vi "Get_Position_Info.vi"(2 "Analysis Info cluster":T1[](array[typedef]) {"Sync Delay Time (s)" format="%.4f"; "Total Meas Time (s)" format="%_5g"; "Sd Error in Variance" format="%_3g"; "Skew_u" format="%_3g"; "% u'/U" format="%_3g"; "Sd Error in Mean" format="%_3g"; "Kurt_u" format="%_3g"; "u^4" format="%_3g"; "u^3" format="%_3g"; "U" format="%_3g"; "u^2" format="%_3g"}, 3 "Setup file string":string) -> (0 "Analysis Info cluster 2":T1[](array[typedef]) {"Sync Delay Time (s)" format="%.4f"; "Total Meas Time (s)" format="%_5g"; "Sd Error in Variance" format="%_3g"; "Skew_u" format="%_3g"; "% u'/U" format="%_3g"; "Sd Error in Mean" format="%_3g"; "Kurt_u" format="%_3g"; "u^4" format="%_3g"; "u^3" format="%_3g"; "U" format="%_3g"; "u^2" format="%_3g"})   [LabVIEW 2021]
uses:
  Controls/Analysis_info_cluster.ctl
  Controls/Inst_type.ctl
  Controls/Instrument_Array.ctl
  Controls/User_Specific_mode.ctl
  Globals/Meas_global.vi
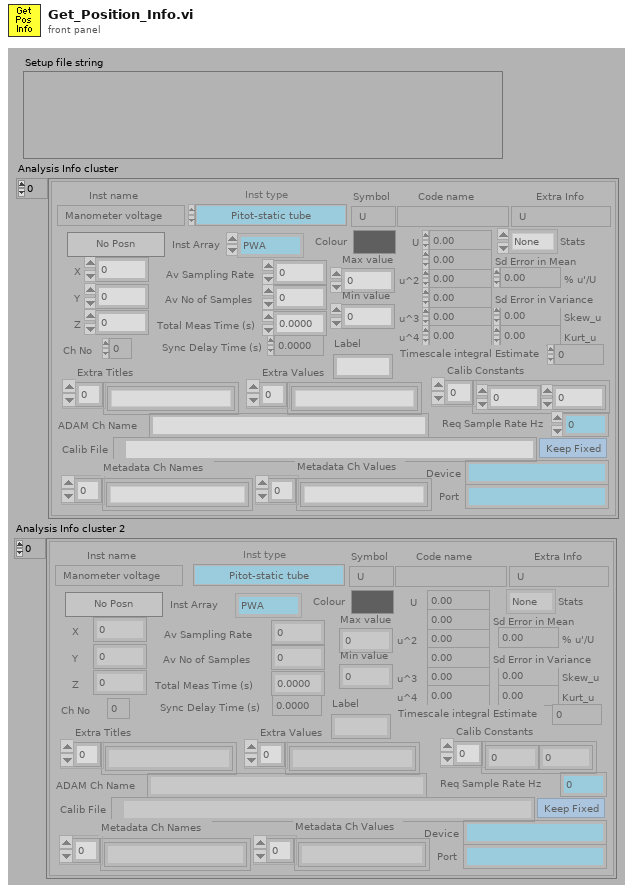
[diagram p1: front panel]
types:
  T1 = typedef "Analysis_info_cluster.ctl" = cluster{"Colour":u32, "Inst type":T2, "Inst name":string, "Symbol":string, "Code name":string, "Extra Info":string, "Inst Array":T3, "Extra Titles":string[], "Extra Values":string[], "U":dbl, "u^2":dbl, "u^3":dbl, "u^4":dbl, "Skew_u":dbl, "Kurt_u":dbl, "Sd Error in Mean":dbl, "% u'/U":dbl, "X":dbl, "Y":dbl, "Z":dbl, "Timescale integral Estimate":dbl, "Sd Error in Variance":dbl, "Calib File":path, "Calib Constants":dbl[], "Output Position":bool, "Stats":enum16{"None", "Basic", "Full"}, "Av Sampling Rate":dbl, "Av No of Samples":dbl, "Total Meas Time (s)":dbl, "ADAM Ch Name":string, "Max value":dbl, "Min value":dbl, "Req Sample Rate Hz":dbl, "Sync Delay Time (s)":dbl, "Ch No":i16, "Device":string, "Use Latest Calib":bool, "Port":string, "Metadata Ch Names":string[], "Metadata Ch Values":string[], "Label":string}
  T2 = typedef "Inst_type.ctl" = enum16{"Raw voltage", "Raw with zero offsetting", "Propeller anemometer", "Pressure Transducer", "Pitot-static tube", "Hot wire", "Cross wire 1", "Cross wire 2", "Generic Linear", "Generic Polynomial", "Generic BackPoly", "Fast FID", "Thermocouple", "Cold wire", "Pulsed Wire", "LDA Vel", "LDA Tran time", "LDA Arr time", "Microphone"}
  T3 = typedef "Instrument_Array.ctl" = enum16{"PWA", "LDA", "Analogue"}
  T4 = typedef "Initial Positions.ctl" = cluster{"Initial XYZ":dbl[], "Traverse Setup":string, "On Axes":string, "Identity String":string}
  T5 = typedef "Post_Process.ctl" = enum16{"Take New Data", "Post Process Raw Data File"}
  T6 = typedef "User_Specific_mode.ctl" = enum16{"Check VI only", "Run VI"}
  T7 = cluster{"Initial XYZ[0]":dbl, "Initial XYZ[1]":dbl, "Initial XYZ[2]":dbl}
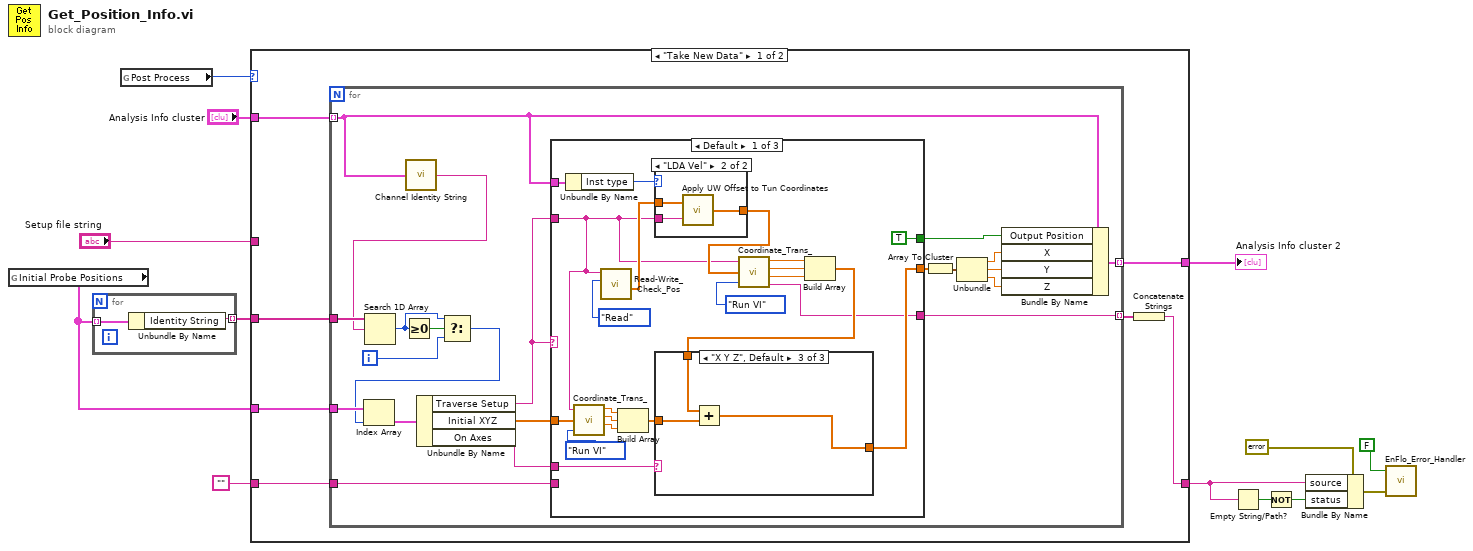
[diagram p0: block diagram]
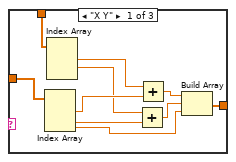
[diagram p3: hidden frame]
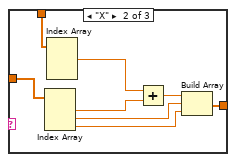
[diagram p4: hidden frame]
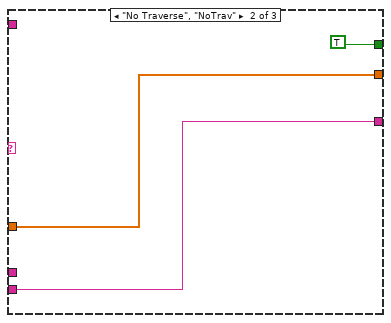
[diagram p5: hidden frame]
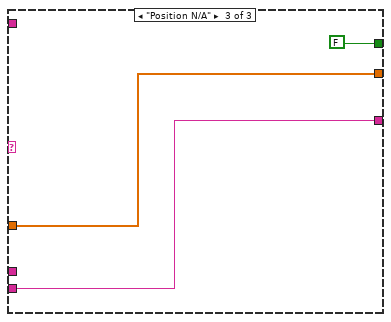
[diagram p6: hidden frame]
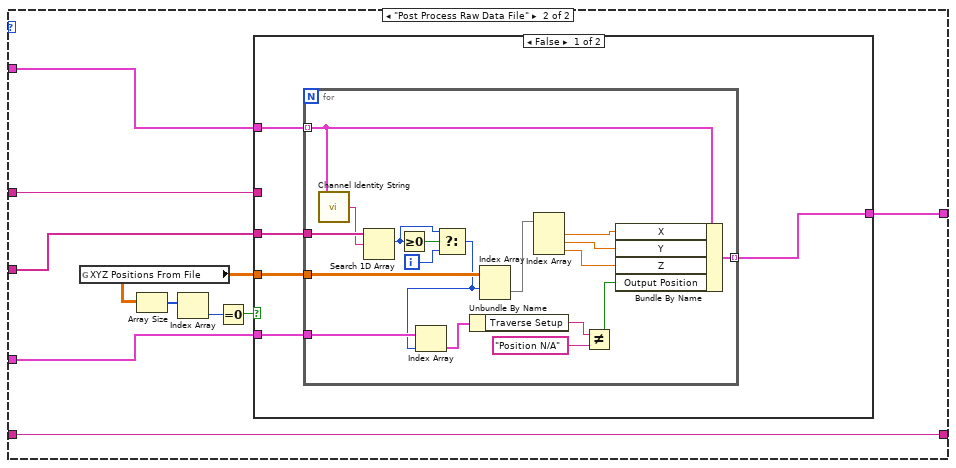
[diagram p7: hidden frame]
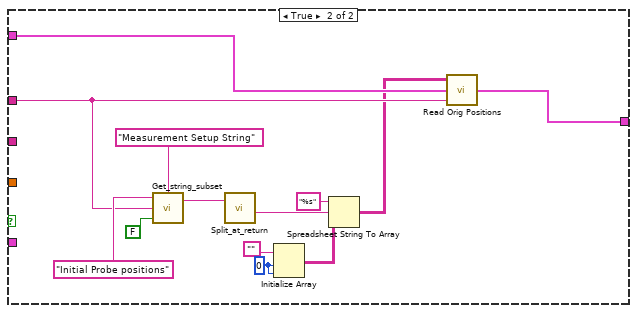
[diagram p8: hidden frame]
diagram:
  n1 = global read "Meas_global.vi" "Initial Probe Positions"() -> (w2:T4[])
  n2 = for {
    tunnel: [w15] -> w1 mode=indexing
    tunnel: w2 -> [w14] mode=indexing
    n3 = Unbundle By Name(w14) -> ("Identity String"=w15:string)
  }
  n4 = global read "Meas_global.vi" "Post Process"() -> (w3:T5)
  n5 = case shown="\"Take New Data\"" w3 {
    tunnel: "Setup file string" -> [_ w104]
    tunnel: "Analysis Info cluster" -> [w22 w105]
    tunnel: [w21 w102] -> w11
    tunnel: [w18 w103] -> w6
    tunnel: "" -> [w20 w103]
    tunnel: w2 -> [w17 w101]
    tunnel: w1 -> [w16 w96]
    frame "Take New Data" {
      n6 = for {
        tunnel: [w38] -> w21 mode=indexing
        tunnel: w22 -> [w28] mode=indexing
        tunnel: [w35] -> w19 mode=indexing
        tunnel: w20 -> [w36]
        tunnel: w17 -> [w34]
        tunnel: w16 -> [w29]
        i -> [w25]
        n7 = call "Channel Identity String.vi"("Analysis Cluster"=w28) -> ("Identity String"=w27:string)
        n8 = Search 1D Array(1D array=w29, element=w27) -> (index of element=w24:i32)  [unwired: 1 out]
        n9 = Greater Or Equal To 0?(x=w24) -> (x >= 0?=w26:bool)
        n10 = Select(t=w24, s=w26, f=w25) -> (s? t:f=w23:i32)
        n11 = Index Array(array=w34, index=w23) -> (element=w33:T4)
        n12 = Unbundle By Name(w33) -> ("Traverse Setup"=w31:string, "Initial XYZ"=w32:dbl[], "On Axes"=w30:string)
        n13 = case shown="Default" w31 {
          tunnel: [w64 w92 w95] -> w43
          tunnel: w32 -> [w49 w92 w95]
          tunnel: w31 -> [w48 _ _]
          tunnel: w30 -> [w57 _ _]
          tunnel: [TRUE TRUE FALSE] -> w37
          tunnel: [w55 w90 w93] -> w35
          tunnel: w36 -> [_ w90 w93]
          tunnel: w28 -> [w53 _ _]
          frame Default {
            n14 = Unbundle By Name(w53) -> ("Inst type"=w52:T2)
            n15 = call "Coordinate_Trans_.vi"("Traverse Name"=w48, "Input Position"=w49, "Simulate/Run"=User_Specific_mode."Run VI") -> ("X"=w47:sgl, "Y"=w46:sgl, "Z"=w45:sgl)  [unwired: 1 out]
            n16 = call "Read-Write_Check_Pos.vi"("Mode"=enum16{"Read", "Write"}."Read", "Traverse Name"=w48) -> ("Position Output"=w54:sgl[])  [unwired: 5 in, 2 out]
            n17 = Build Array(w47, w46, w45) -> (w44:sgl[])
            n18 = case shown="\"LDA Vel\"" w52 {
              tunnel: w54 -> [w65 w68]
              tunnel: w48 -> [_ w67]
              tunnel: [w65 w66] -> w51
              frame Default {
              }
              frame "LDA Vel" {
                n19 = call "Apply UW Offset to Tun Coordinates.vi"("Traverse Name"=w67, "Tunnel Coordinates"=w68) -> ("UW Offset Applied"=w66:sgl[])
              }
            }
            n20 = call "Coordinate_Trans_.vi"("Traverse Name"=w48, "Input Position"=w51, "Simulate/Run"=User_Specific_mode."Run VI") -> ("X"=w63:sgl, "Y"=w62:sgl, "Z"=w61:sgl, "Error String"=w55:string)
            n21 = Build Array(w63, w62, w61) -> (w60:sgl[])
            n22 = case shown="\"X Y Z\", Default" w57 {
              tunnel: w44 -> [w78 w86 w89]
              tunnel: [w74 w82 w88] -> w64
              tunnel: w60 -> [w77 w85 w87]
              frame "X Y" {
                n23 = Index Array(array=w78) -> (element #1=w75:sgl, element #2=w71:sgl, element #3=w69:sgl)  [unwired: 3 in]
                n24 = Index Array(array=w77) -> (element #1=w76:sgl, element #2=w72:sgl)  [unwired: 3 in, 1 out]
                n25 = Add(x=w72, y=w71) -> (x+y=w70:sgl)
                n26 = Add(x=w76, y=w75) -> (x+y=w73:sgl)
                n27 = Build Array(w73, w70, w69) -> (w74:sgl[])
              }
              frame "X" {
                n28 = Index Array(array=w86) -> (element #1=w83:sgl, element #2=w79:sgl, element #3=w80:sgl)  [unwired: 3 in]
                n29 = Index Array(array=w85) -> (element #1=w84:sgl)  [unwired: 3 in, 2 out]
                n30 = Add(x=w84, y=w83) -> (x+y=w81:sgl)
                n31 = Build Array(w81, w79, w80) -> (w82:sgl[])
              }
              frame "X Y Z", Default {
                n32 = Add(x=w87, y=w89) -> (x+y=w88:sgl[])
              }
            }
          }
          frame "No Traverse", "NoTrav" {
          }
          frame "Position N/A" {
          }
        }
        n33 = Array To Cluster(array=w43) -> (cluster=w42:T7)
        n34 = Unbundle(w42) -> ("Initial XYZ[0]"=w41:dbl, "Initial XYZ[1]"=w40:dbl, "Initial XYZ[2]"=w39:dbl)
        n35 = Bundle By Name(cluster=w28, "Output Position"=w37, "X"=w41, "Y"=w40, "Z"=w39) -> (w38:T1)
      }
      n36 = Concatenate Strings(w19) -> (w18:string)
    }
    frame "Post Process Raw Data File" {
      n37 = global read "Meas_global.vi" "XYZ Positions From File"() -> (w100:dbl[][])
      n38 = Array Size(array=w100) -> (size(s)=w99:i32[])
      n39 = Index Array(array=w99) -> (element=w98:i32)  [unwired: 1 in]
      n40 = Equal To 0?(x=w98) -> (x = 0?=w97:bool)
      n41 = case shown="False" w97 {
        tunnel: w105 -> [w110 w141]
        tunnel: w104 -> [_ w130]
        tunnel: [w109 w140] -> w102
        tunnel: w101 -> [w108 _]
        tunnel: w100 -> [w107 _]
        tunnel: w96 -> [w106 _]
        frame False {
          n42 = for {
            tunnel: w110 -> [w116] mode=indexing
            tunnel: [w124] -> w109 mode=indexing
            tunnel: w108 -> [w123]
            tunnel: w107 -> [w118]
            tunnel: w106 -> [w117]
            i -> [w112]
            n43 = call "Channel Identity String.vi"("Analysis Cluster"=w116) -> ("Identity String"=w115:string)
            n44 = Search 1D Array(1D array=w117, element=w115) -> (index of element=w111:i32)  [unwired: 1 out]
            n45 = Greater Or Equal To 0?(x=w111) -> (x >= 0?=w114:bool)
            n46 = Select(t=w111, s=w114, f=w112) -> (s? t:f=w113:i32)
            n47 = Index Array(array=w123, index=w113) -> (element=w122:T4)
            n48 = Unbundle By Name(w122) -> ("Traverse Setup"=w120:string)
            n49 = Index Array(array=w118, index (row)=w113) -> (element=w128:dbl[])  [unwired: 1 in]
            n50 = Index Array(array=w128) -> (element #1=w127:dbl, element #2=w126:dbl, element #3=w125:dbl)  [unwired: 3 in]
            n51 = Not Equal?(x=w120, y="Position N/A") -> (x != y?=w119:bool)
            n52 = Bundle By Name(cluster=w116, "X"=w127, "Y"=w126, "Z"=w125, "Output Position"=w119) -> (w124:T1)
          }
        }
        frame True {
          w137 = 0 ("Dimension Size")
          n53 = call "Get_string_subset.vi"("String Name"="Measurement Setup String", "Show Dialog?"=FALSE, "String to split"=w130, "File Label"="Initial Probe positions") -> ("Output string"=w139:string)  [unwired: 1 out]
          n54 = call "Split_at_return.vi"("String"=w139) -> ("after substring"=w134:string)  [unwired: 1 in, 3 out]
          n55 = Initialize Array("", w137, w137) -> (w138:string[][])
          n56 = Spreadsheet String To Array(format string="%s", spreadsheet string=w134, array type (2D Dbl)=w138) -> (array=w129:string[][])  [unwired: 1 out]
          n57 = call "Read Orig Positions.vi"("Setup file string"=w130, "Analysis Info cluster In"=w141, "Array in"=w129) -> ("Analysis Info cluster Out"=w140:T1[])  [unwired: 2 in]
        }
      }
    }
  }
  "Analysis Info cluster 2" <- w11
  n58 = Empty String/Path?(string/path=w6) -> (empty?=w8:bool)
  n59 = Not(x=w8) -> (.not. x?=w7:bool)
  n60 = Bundle By Name(cluster=errorcluster {"status"=FALSE, "code"=0, "source"=""} ("error in (no error)"), "source"=w6, "status"=w7) -> (w5:errorcluster)
  n61 = call "EnFlo_Error_Handler.vi"("error in (no error)"=w5, "Dialog Box (F)"=FALSE ("Dialog Box (T)")) -> ()  [unwired: 2 in, 2 out]
